vi "3.6 .vi"() -> ()   [LabVIEW 2019]
uses:
  <vilib>/Analysis/NI_AALBase.lvlib
panel:
  out "Waveform Graph 2":dbl[](graph)
  in  "N":dbl
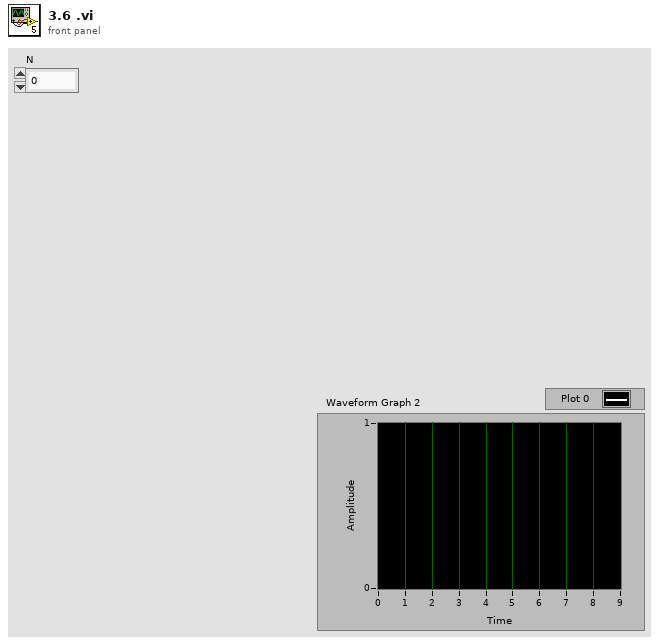
[diagram p1: front panel]
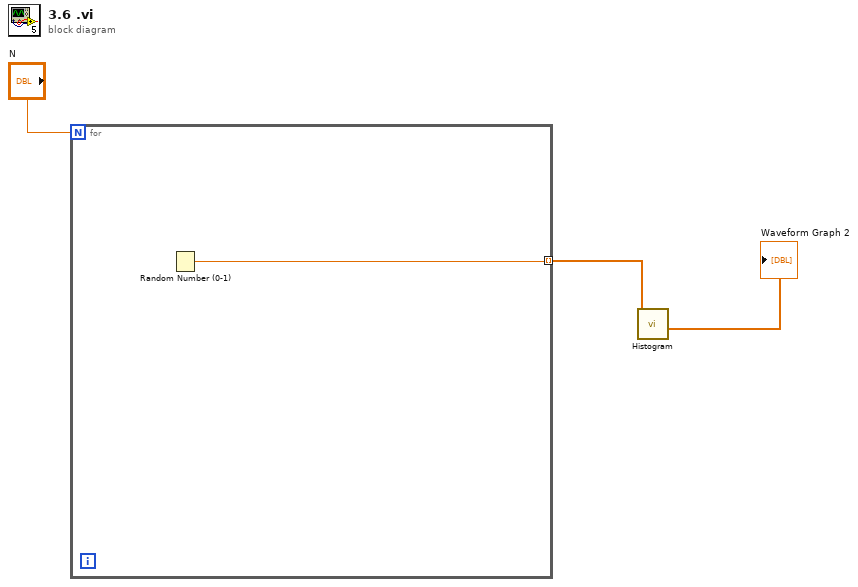
[diagram p0: block diagram]
diagram:
  n1 = for {
    N: "N" -> [_]
    tunnel: [w4] -> w2 mode=indexing
    n2 = Random Number (0-1)() -> (number: 0 to 1=w4:dbl)
  }
  n3 = call <vilib>:"Histogram.vi"("X"=w2) -> ("X Values"=→"Waveform Graph 2":dbl[])  [unwired: 7 in, 3 out]
